vi "GetParametersDialog.vi"(9 "Main VI Ref":refnum<vi>) -> (0 "Error Out":errorcluster, 2 "MainData":T1)   [LabVIEW 2020]
doc: "Gets the basic parameters needed to create a main board and set up game rules."
uses:
  Ctrls/MainData.ctl
panel:
  in  "OK":bool
  in  "Size":i32(slide)=40 min=0 max=70 step=5 scale=10.0..70.0
  in  "Rule":string="23/3"
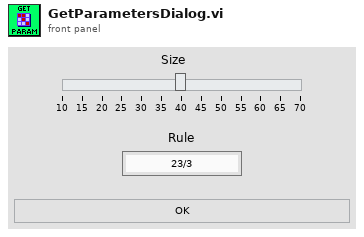
[diagram p1: front panel]
types:
  T1 = typedef "MainData.ctl" = cluster{"Size":i32, "Live rule":i32[], "Dead rule":i32[]}
  T2 = enum32{"Invalid", "Standard", "Closed", "Hidden", "Minimized", "Maximized"}
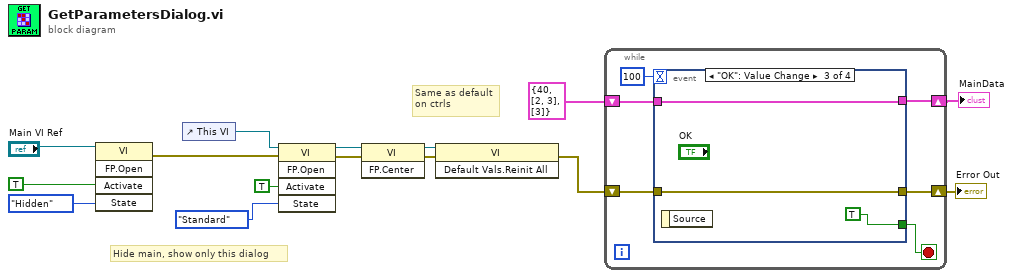
[diagram p0: block diagram]
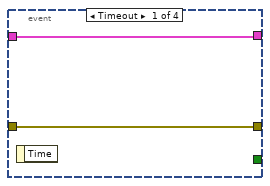
[diagram p2: hidden frame]
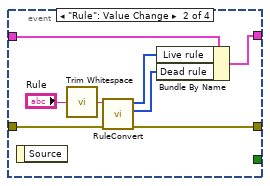
[diagram p3: hidden frame]
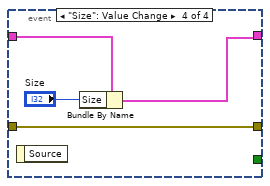
[diagram p4: hidden frame]
diagram:
  # "Same as default\non ctrls"
  # "Hide main, show only this dialog"
  n1 = invoke class="VI" method="FP.Open"(reference="Main VI Ref", "Activate"=TRUE ("Activate?"), "State"=T2."Hidden") -> (error out=w3:errorcluster)  [unwired: 2 in, 4 out]
  n2 = control-ref of="This VI"() -> (w12:refnum<vi>)
  n3 = invoke class="VI" method="FP.Open"(reference=w12, error in=w3, "Activate"=TRUE ("Activate?"), "State"=T2."Standard") -> (reference out=w9:refnum<vi>, error out=w8:errorcluster)  [unwired: 1 in, 3 out]
  n4 = invoke class="VI" method="FP.Center"(reference=w9, error in=w8) -> (reference out=w1:refnum<vi>, error out=w7:errorcluster)  [unwired: 1 in, 1 out]
  n5 = invoke class="VI" method="Default Vals.Reinit All"(reference=w1, error in=w7) -> (error out=w2:errorcluster)  [unwired: 1 in, 2 out]
  n6 = while {
    shift-right: [w18] -> w14
    shift-left: T1 {"Size"=40, "Live rule"=[2, 3], "Dead rule"=[3]} ("output cluster 2") -> [w19]
    shift-right: [w20] -> w13
    shift-left: w2 -> [w21]
    stop <- w16 stop-if-true
    n7 = event shown="[2] \"OK\": Value Change" {
      selector: _ -> [_ _ _ _]
      dyn-events: _ -> [_ _ _ _]
      timeout: 100 -> [_ _ _ _]
      tunnel: w21 -> [w23 w30 w33 w38]
      tunnel: [w23 w29 w33 w38] -> w20
      tunnel: w19 -> [w22 w28 w32 w37]
      tunnel: [w22 w25 w32 w35] -> w18
      tunnel: [_ _ TRUE _] -> w16
      event Timeout {
        n8 = event-data() -> ()  [unwired: 1 in, 1 out]
      }
      event "Rule": Value Change {
        n9 = event-data() -> ()  [unwired: 1 in, 1 out]
        n10 = call <vilib>:"Trim Whitespace.vi"("string"="Rule") -> ("trimmed string"=w24:string)  [unwired: 1 in]
        n11 = call "RuleConvert.vi"("Error In"=w30, "String"=w24) -> ("Error Out"=w29:errorcluster, "Dead rule"=w26:i32[], "Live rule"=w27:i32[])  [unwired: 7 in]
        n12 = Bundle By Name(cluster=w28, "Live rule"=w27, "Dead rule"=w26) -> (w25:T1)
      }
      event "OK": Value Change {
        n13 = event-data() -> ()  [unwired: 1 in, 1 out]
      }
      event "Size": Value Change {
        n14 = event-data() -> ()  [unwired: 1 in, 1 out]
        n15 = Bundle By Name(cluster=w37, "Size"="Size") -> (w35:T1)
      }
    }
  }
  "MainData" <- w14
  "Error Out" <- w13
